vi "runSender.vi"(8 "error in (no error)":errorcluster, 10 "ScriptEvent":refnum<class "ScriptEvent.lvclass">, 11 "sender in":refnum<class "sender.lvclass">) -> (0 "error out":errorcluster, 3 "sender out":refnum<class "sender.lvclass">)   [LabVIEW 2009, in "Events.lvlib" / "sender.lvclass"]
uses:
  sender.lvclass
  ScriptEvent.lvclass
panel:
  in  "sendClose":bool
  in  "sendSave":bool
  in  "sendOpen":bool
  in  "Path":path
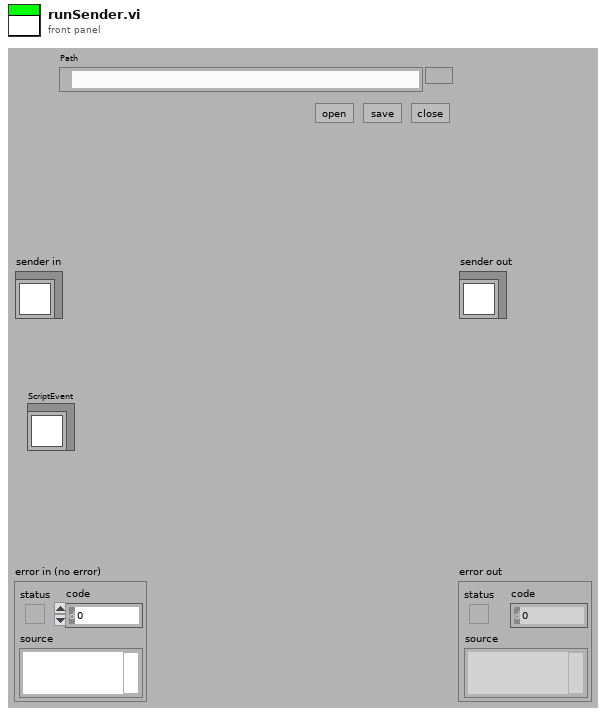
[diagram p1: front panel]
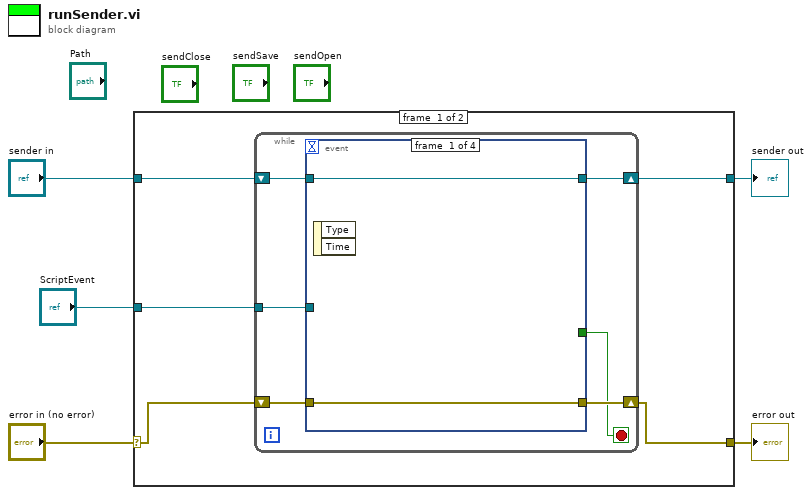
[diagram p0: block diagram]
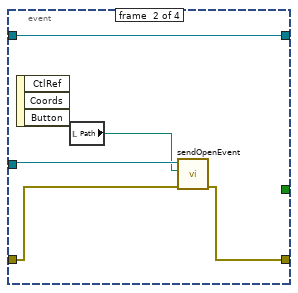
[diagram p2: hidden frame]
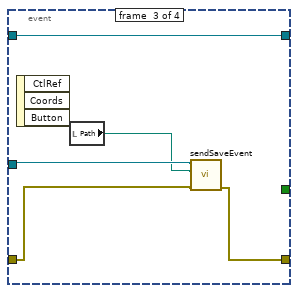
[diagram p3: hidden frame]
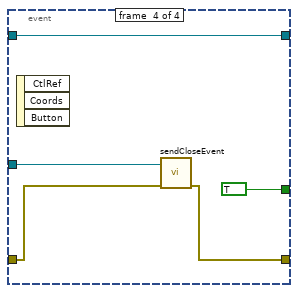
[diagram p4: hidden frame]
diagram:
  n1 = case shown="No Error" "error in (no error)" {
    selector: "error in (no error)" -> [w10 w35]
    tunnel: [w7 w35] -> w4
    tunnel: [w8 w34] -> w2
    tunnel: "sender in" -> [w9 w34]
    tunnel: "ScriptEvent" -> [w6 _]
    frame #0 {
      n2 = while {
        shift-right: [w15] -> w8
        shift-left: w9 -> [w16]
        shift-right: [w13] -> w7
        shift-left: w10 -> [w14]
        tunnel: w6 -> [w12]
        stop <- w11 stop-if-true
        n3 = event shown="[3] \"sendClose\": Mouse Down" {
          selector: _ -> [_ _ _ _]
          dyn-events: _ -> [_ _ _ _]
          timeout: _ -> [_ _ _ _]
          tunnel: w16 -> [w18 w23 w28 w33]
          tunnel: [w18 w23 w28 w33] -> w15
          tunnel: w12 -> [_ w22 w27 w32]
          tunnel: w14 -> [w17 w20 w25 w31]
          tunnel: [w17 w19 w24 w30] -> w13
          tunnel: [_ _ _ TRUE] -> w11
          event #0 {
            n4 = event-data() -> ()  [unwired: 1 in, 2 out]
          }
          event #1 {
            n5 = event-data() -> ()  [unwired: 1 in, 3 out]
            n6 = local read "Path"() -> (w21:path)
            n7 = call "sendOpenEvent.vi"("error in (no error)"=w20, "Path"=w21, "ScriptEvent in"=w22) -> ("error out"=w19:errorcluster)  [unwired: 7 in, 1 out]
          }
          event #2 {
            n8 = event-data() -> ()  [unwired: 1 in, 3 out]
            n9 = local read "Path"() -> (w26:path)
            n10 = call "sendSaveEvent.vi"("error in (no error)"=w25, "Path"=w26, "ScriptEvent in"=w27) -> ("error out"=w24:errorcluster)  [unwired: 7 in, 1 out]
          }
          event #3 {
            n11 = event-data() -> ()  [unwired: 1 in, 3 out]
            n12 = call "sendCloseEvent.vi"("error in (no error)"=w31, "ScriptEvent in"=w32) -> ("error out"=w30:errorcluster)  [unwired: 8 in, 1 out]
          }
        }
      }
    }
    frame #1 {
    }
  }
  "error out" <- w4
  "sender out" <- w2
